vi "overlap.vi"(4 "Cluster":cluster{"Numeric":dbl, "Numeric 2":dbl}, 5 "Array":cluster{"Numeric":dbl, "Numeric 2":dbl}[](array[cluster])) -> (0 "Boolean":bool, 1 "Numeric":i32, 2 "Cluster 2":cluster{"Numeric":dbl, "Numeric 2":dbl})   [LabVIEW 2014]
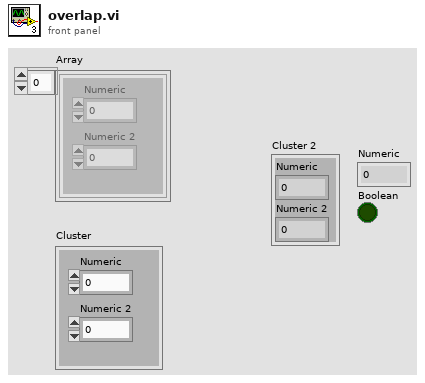
[diagram p1: front panel]
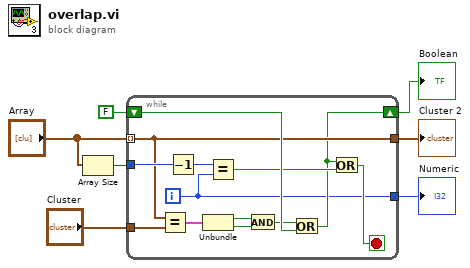
[diagram p0: block diagram]
diagram:
  n1 = Array Size(array="Array") -> (size(s)=w7:i32)
  n2 = while {
    tunnel: "Array" -> [w11] mode=indexing
    tunnel: "Cluster" -> [w20]
    shift-right: [w9] -> w4
    shift-left: FALSE -> [w19]
    tunnel: w7 -> [w14]
    tunnel: [w11] -> w1
    tunnel: [w8] -> w5
    i -> [w8]
    stop <- w10 stop-if-true
    n3 = Equal?(x=w11, y=w20) -> (x = y?=w18:cluster{"Numeric":bool, "Numeric 2":bool})
    n4 = Decrement(x=w14) -> (x-1=w13:i32)
    n5 = Unbundle(w18) -> ("Numeric"=w17:bool, "Numeric 2"=w16:bool)
    n6 = Equal?(x=w13, y=w8) -> (x = y?=w12:bool)
    n7 = And(x=w17, y=w16) -> (x .and. y?=w15:bool)
    n8 = Or(x=w15, y=w19) -> (x .or. y?=w9:bool)
    n9 = Or(x=w9, y=w12) -> (x .or. y?=w10:bool)
  }
  "Numeric" <- w5
  "Boolean" <- w4
  "Cluster 2" <- w1
